vi "GUI FFT Calc From Waves.vi"(2 "graphs count (2)":i32=2, 4 "source mode":T1, 5 "max size":T4=enum."1 MSa" caption="Limit waveform size", 6 "sub-rec index ref":refnum<vi>, 7 "window type":T3, 8 "error in (no error)":errorcluster, 9 "phase ref":refnum<vi>, 10 "rec index ref":refnum<vi>, 11 "record info":T5={"header path"=path "", "group id"=0, "average id"=0, "Time Stamp"=timestamp(0 s since 1904-01-01), "max samples"=0, "first sample"=0, "first smpl [%]"=-1.0, "kill viewer"=FALSE}) -> (0 "error out":errorcluster, 3 "waveforms":T2[](array[typedef]))   [LabVIEW 2020]
doc: "Fetch measurement session, calculate FFTs from waveforms directly, prepare up to 2 graphs for display. Also fill in phase/wave selectors."
uses:
  GUI Waveform Info.ctl
  GUI FFT Limit Samples.ctl
  other/fftw3/source/window/Window Type.ctl
  processing/QWTB/Meas Proc QWTB Spectrum Data.ctl
  files/Meas Sample Reader Source Mode.ctl
  other/fftw3/source/FFTWDLL.lvlib
panel:
  in  "grp index":u16(ring) items=["Last", "Group 1"]
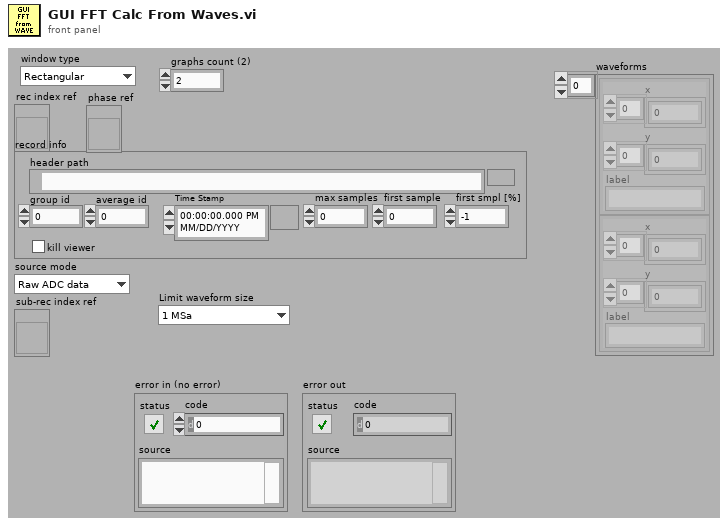
[diagram p1: front panel]
types:
  T1 = typedef "Meas Sample Reader Source Mode.ctl" = enum16{"Raw ADC data", "Transducers"}
  T2 = typedef "Meas Proc QWTB Spectrum Data.ctl" = cluster{"x":sgl[], "y":sgl[], "label":string}
  T3 = typedef "FFTWDLL.lvlib/Window Type.ctl" = enum16{"Rectangular", "Hanning", "Blackman-Harris", "Flattop 248D"}
  T4 = typedef "GUI FFT Limit Samples.ctl" = enum16{"16 kSa", "32 kSa", "64 kSa", "128 kSa", "256 kSa", "512 kSa", "1 MSa", "2 MSa", "4 MSa", "8 MSa", "16 MSa"}
  T5 = typedef "GUI Waveform Info.ctl" = cluster{"header path":path, "group id":i32, "average id":i32, "Time Stamp":timestamp, "max samples":i64, "first sample":i64, "first smpl [%]":dbl, "kill viewer":bool}
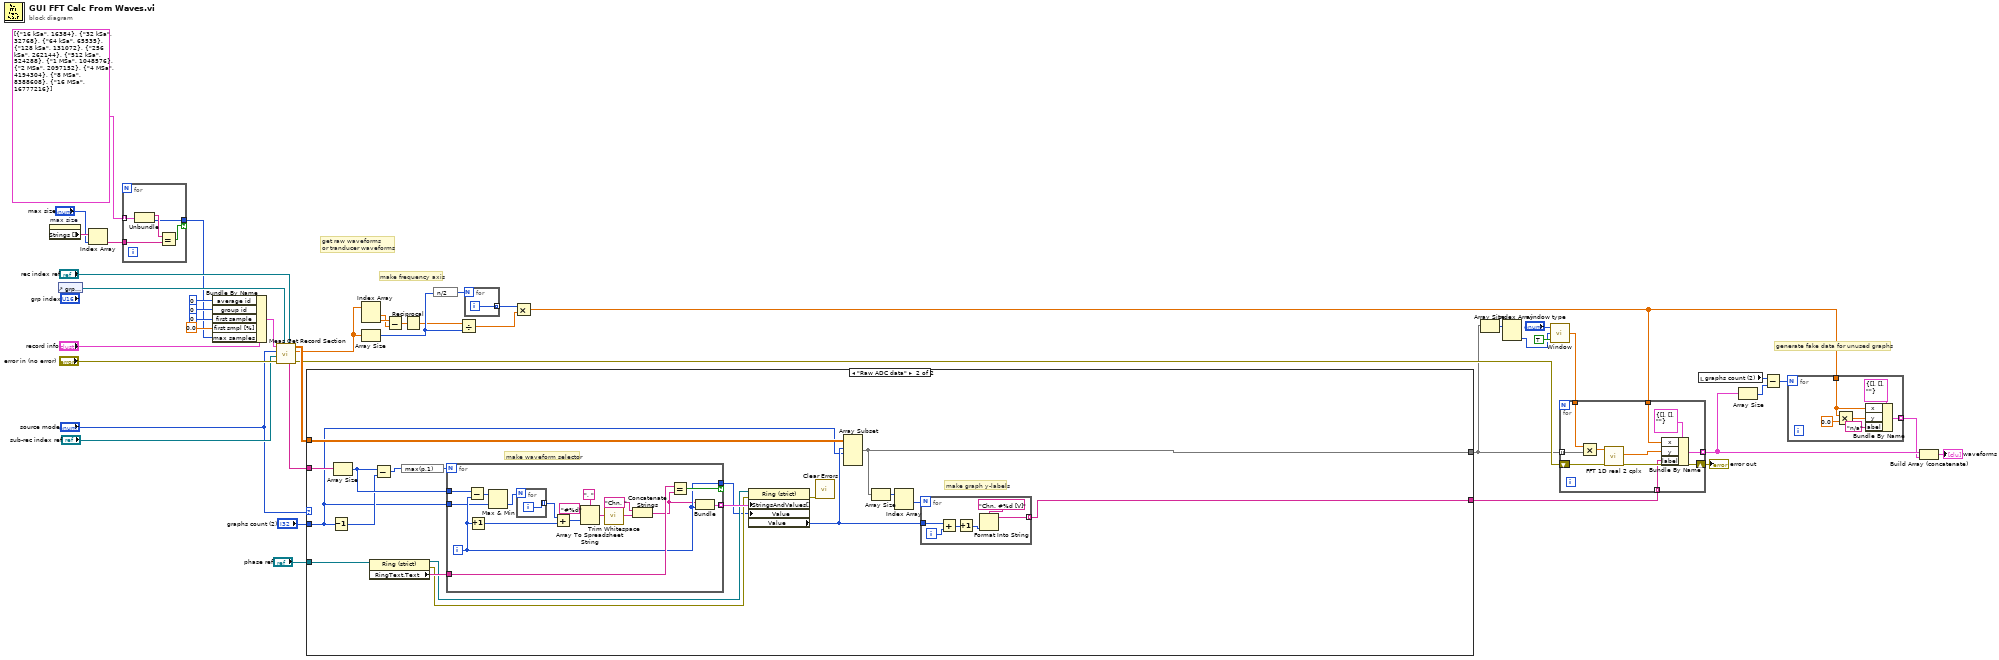
[diagram p0: block diagram]
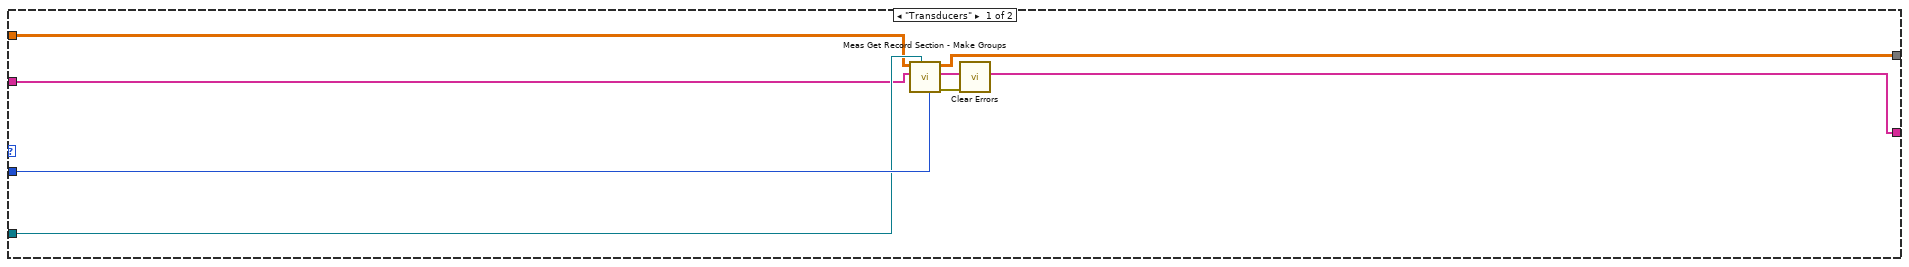
[diagram p2: hidden frame]
diagram:
  # "generate fake data for unused graphs"
  # "make frequency axis"
  # "get raw waveforms\nor tranducer waveforms"
  n1 = property on="max size" class="Enum (strict)"() -> ("Strings []"=w42:string[])  [unwired: 2 in, 2 out]
  n2 = control-ref of="grp index"() -> (w44:refnum<vi>)
  n3 = Index Array(array=w42, index="max size") -> (element=w3:string)
  n4 = for {
    tunnel: w3 -> [w49]
    tunnel: cluster{string, i64}[] [{"16 kSa", 16384}, {"32 kSa", 32768}, {"64 kSa", 65535}, {"128 kSa", 131072}, {"256 kSa", 262144}, {"512 kSa", 524288}, {"1 MSa", 1048576}, {"2 MSa", 2097152}, {"4 MSa", 4194304}, {"8 MSa", 8388608}, {"16 MSa", 16777216}] -> [w50] mode=indexing
    tunnel: [w47] -> w1 if=w46
    n5 = Unbundle(w50) -> (w48:string, w47:i64)
    n6 = Equal?(x=w48, y=w49) -> (x = y?=w46:bool)
  }
  n7 = Bundle By Name(cluster="record info", "average id"=0, "group id"=0, "first sample"=i64 0, "first smpl [%]"=0.0, "max samples"=w1) -> (w40:T5)
  n8 = call "Meas Get Record Section.vi"("record index ref"="rec index ref", "grp index ref"=w44, "error in"="error in (no error)", "sub-rec index ref"="sub-rec index ref", "source mode"="source mode", "record info"=w40) -> ("error out"=w25:errorcluster, "time [s]"=w30:dbl[], "waveforms [V]"=w36:sgl[][], "labels"=w18:string[])  [unwired: 1 in, 1 out]
  n9 = case shown="\"Raw ADC data\"" "source mode" {
    tunnel: w36 -> [w53 w69]
    tunnel: [w57 w60] -> w13
    tunnel: w18 -> [w52 w67]
    tunnel: [w56 w59] -> w17
    tunnel: "phase ref" -> [w54 w66]
    tunnel: "graphs count (2)" -> [w55 w58]
    frame "Transducers" {
      n10 = call "Meas Get Record Section - Make Groups.vi"("max group size (2)"=w55, "waveforms group selector ref"=w54, "all labels"=w52, "all waveforms in [V]"=w53) -> ("error out"=w51:errorcluster, "selected labels"=w56:string[], "selected waveforms out [V]"=w57:sgl[][])  [unwired: 4 in, 1 out]
      n11 = call <vilib>:"Clear Errors.vi"("error in (no error)"=w51) -> ()  [unwired: 5 in, 2 out]
    }
    frame "Raw ADC data" {
      # "make graph y-labels"
      # "make waveform selector"
      n12 = Decrement(x=w58) -> (x-1=w63:i32)
      n13 = Array Size(array=w67) -> (size(s)=w65:i32)
      n14 = property class="Ring (strict)"(reference=w66) -> (reference out=w72:refnum<vi>, error out=w73:errorcluster, "RingText.Text"=w75:string)  [unwired: 1 in]
      n15 = Subtract(x=w65, y=w63) -> (x-y=w64:i32)
      n16 = expression code="max(p,1)"(w64) -> (w76:i32)
      n17 = for {
        N: w76 -> [_]
        tunnel: w65 -> [w99]
        tunnel: [w98] -> w74 mode=indexing
        tunnel: w75 -> [w97]
        tunnel: [w95] -> w71 if=w96
        tunnel: w58 -> [w84]
        i -> [w95]
        n18 = Subtract(x=w99, y=w95) -> (x-y=w85:i32)
        n19 = Increment(x=w95) -> (x+1=w93:i32)
        n20 = Max & Min(x=w85, y=w84) -> (min(x,y)=w83:i32)  [unwired: 1 out]
        n21 = for {
          N: w83 -> [_]
          tunnel: [w100] -> w94 mode=indexing
          i -> [w100]
        }
        n22 = Add(x=w94, y=w93) -> (x+y=w92:i32[])
        n23 = Array To Spreadsheet String(delimiter (Tab)=", ", array=w92, 3:"#%d" ("format string")) -> (spreadsheet string=w89:string)
        n24 = call <vilib>:"Trim Whitespace.vi"("string"=w89) -> ("trimmed string"=w88:string)  [unwired: 1 in]
        n25 = Concatenate Strings("Chn. " ("string"), w88) -> (w87:string)
        n26 = Equal?(x=w97, y=w87) -> (x = y?=w96:bool)
        n27 = Bundle(w87, w95) -> (w98:cluster{string, i32})  [unwired: 1 in]
      }
      n28 = property class="Ring (strict)"(reference=w72, error in=w73, "StringsAndValues[]"=w74, "Value"=w71) -> (error out=w70:errorcluster, "Value"=w61:u16)  [unwired: 1 out]
      n29 = call <vilib>:"Clear Errors.vi"("error in (no error)"=w70) -> ()  [unwired: 5 in, 2 out]
      n30 = Array Subset(array=w69, index (row)=w61, length (row)=w58) -> (w60:sgl[][])  [unwired: 2 in]
      n31 = Array Size(array=w60) -> (size(s)=w68:i32[])
      n32 = Index Array(array=w68) -> (element #1=w62:i32)  [unwired: 2 in, 1 out]
      n33 = for {
        N: w62 -> [_]
        tunnel: w61 -> [w81]
        tunnel: [w77] -> w59 mode=indexing
        i -> [w82]
        n34 = Add(x=w81, y=w82) -> (x+y=w80:i32)
        n35 = Increment(x=w80) -> (x+1=w78:i32)
        n36 = Format Into String(format string="Chn. #%d [V]", w78) -> (resulting string=w77:string)  [unwired: 2 in, 1 out]
      }
    }
  }
  n37 = Array Size(array=w30) -> (size(s)=w28:i32)
  n38 = Index Array(array=w30) -> (element #1=w31:dbl, element #2=w32:dbl)  [unwired: 2 in]
  n39 = Subtract(x=w32, y=w31) -> (x-y=w29:dbl)
  n40 = Reciprocal(x=w29) -> (1/x=w23:dbl)
  n41 = expression code="n/2"(w28) -> (w22:i32)
  n42 = Divide(x=w23, y=w28) -> (x/y=w26:dbl)
  n43 = for {
    N: w22 -> [_]
    tunnel: [w101] -> w27 mode=indexing
    i -> [w101]
  }
  n44 = Multiply(x=w27, y=w26) -> (x*y=w7:dbl[])
  n45 = Array Size(array=w13) -> (size(s)=w16:i32[])
  n46 = Index Array(array=w16) -> (element #2=w12:i32)  [unwired: 2 in, 1 out]
  n47 = call "Window.vi"("Normalize? (False)"=TRUE, "N"=w12, "window type"="window type") -> ("window"=w33:dbl[])
  n48 = for {
    tunnel: w13 -> [w111] mode=indexing
    tunnel: w33 -> [w110]
    tunnel: w7 -> [w109]
    tunnel: [w108] -> w6 mode=indexing
    shift-right: [w105] -> w24
    shift-left: w25 -> [w106]
    tunnel: w17 -> [w102] mode=indexing
    n49 = Multiply(x=w110, y=w111) -> (x*y=w107:dbl[])
    n50 = call "FFT 1D real 2 cplx.vi"("error in (no error)"=w106, "y"=w107) -> ("error out"=w105:errorcluster, "amp(Y)"=w104:dbl[])  [unwired: 6 in, 2 out]
    n51 = Bundle By Name(cluster=T2 {"x"=[], "y"=[], "label"=""}, "x"=w109, "y"=w104, "label"=w102) -> (w108:T2)
  }
  "error out" <- w24
  n52 = local read "graphs count (2)"() -> (w10:i32)
  n53 = Array Size(array=w6) -> (size(s)=w9:i32)
  n54 = Subtract(x=w10, y=w9) -> (x-y=w8:i32)
  n55 = for {
    N: w8 -> [_]
    tunnel: w7 -> [w116]
    tunnel: [w112] -> w5 mode=indexing
    n56 = Multiply(x=w116, y=sgl 0.0) -> (x*y=w115:dbl[])
    n57 = Bundle By Name(cluster=T2 {"x"=[], "y"=[], "label"=""}, "x"=w116, "y"=w115, "label"="n/a") -> (w112:T2)
  }
  n58 = Build Array (concatenate)(w6, w5) -> (→"waveforms":T2[])
